vi "Delete Duplicates From 1D-Array (String).vi"(11 "Array in":string[](array[string])) -> (3 "Array w/out dupes out":string[](array[string]))   [LabVIEW 2014, in "hse-misc.lvlib"]
doc: "(v0.2.1b; 2017-08-14 16:44)\n\n\n\n____\nHAMPEL SOFTWARE ENGINEERING v0.7.0 (2018-07-16 18:12)"
uses:
  hse-misc.lvlib
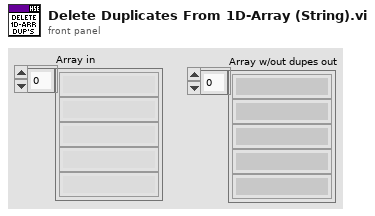
[diagram p1: front panel]
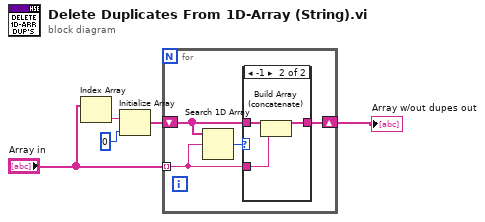
[diagram p0: block diagram]
diagram:
  n1 = Index Array(array="Array in") -> (element=w3:string)  [unwired: 1 in]
  n2 = Initialize Array(w3, 0 ("Dimension Size")) -> (w4:string[])
  n3 = for {
    tunnel: "Array in" -> [w8] mode=indexing
    shift-right: [w7] -> w1
    shift-left: w4 -> [w6]
    n4 = Search 1D Array(1D array=w6, element=w8) -> (index of element=w9:i32)  [unwired: 1 in]
    n5 = case shown="-1" w9 {
      tunnel: w8 -> [_ w13]
      tunnel: [w10 w11] -> w7
      tunnel: w6 -> [w10 w12]
      frame Default {
      }
      frame -1 {
        n6 = Build Array (concatenate)(w12, w13) -> (w11:string[])
      }
    }
  }
  "Array w/out dupes out" <- w1
